vi "IniScrewPara.vi"(8 "error in":errorcluster, 10 "Screw section":string="Info", 11 "INI file path":path=path "D:/ZDX201 塗膠螺絲鎖固自動化_鴻海/ZDX201_LabView/iniData/screw_iniData.ini") -> (0 "data path":path, 1 "Delay":u32, 2 "Screw_L":string="172.100.1.1:1239", 3 "Screw_R":string="172.100.1.22")   [LabVIEW 2019]
uses:
  <vilib>/Utility/config.llb/Read Key (String).vi
  <vilib>/Utility/config.llb/Read Key (U32).vi
  <vilib>/Utility/config.llb/Read Key (Path).vi
  <vilib>/Utility/config.llb/NI_LVConfig.lvlib
panel:
  out "error out":errorcluster
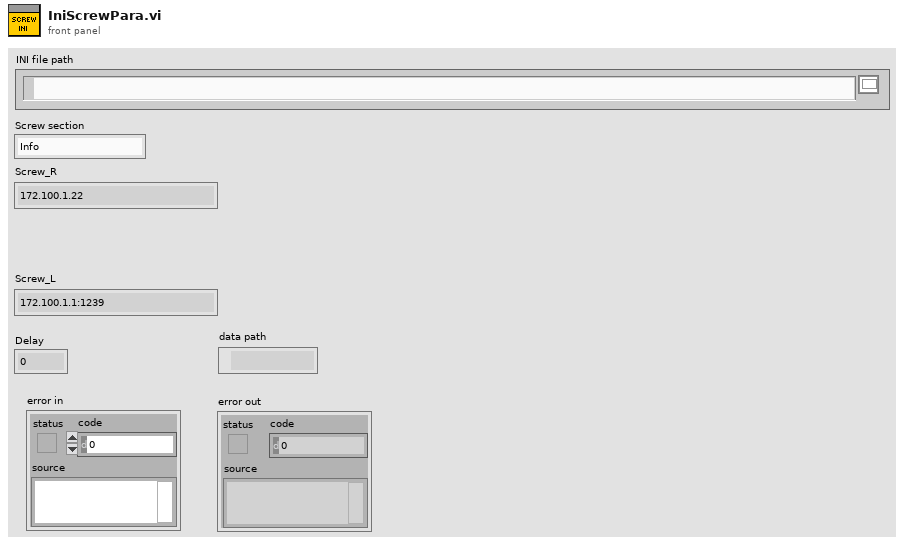
[diagram p1: front panel]
types:
  T1 = typedef "NI_LVConfig.lvlib/Config Data RefNum.ctl" = refnum<k1>
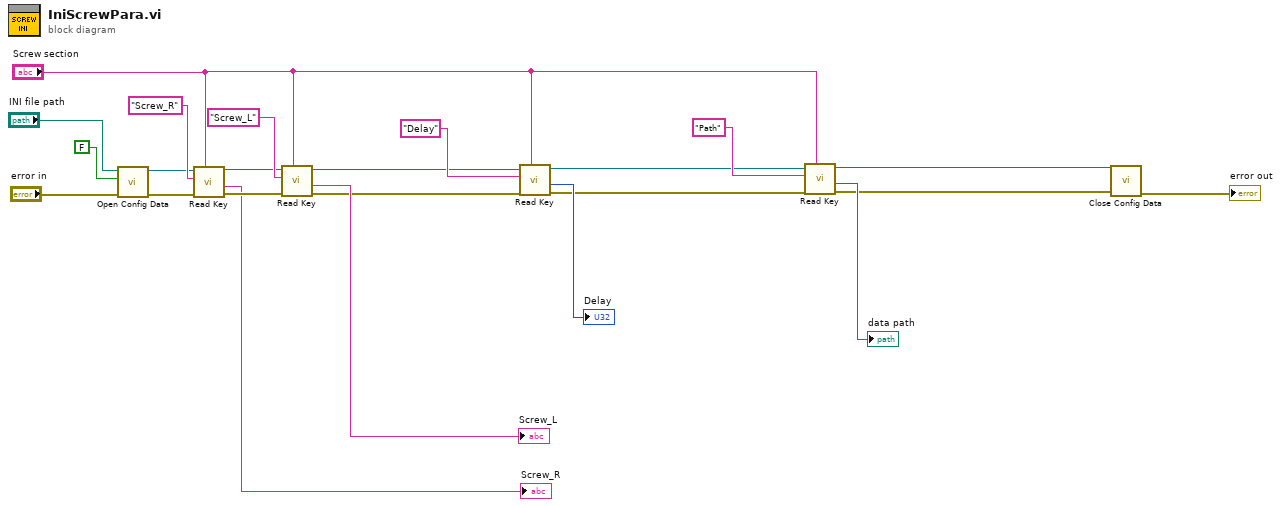
[diagram p0: block diagram]
diagram:
  n1 = call <vilib>:"Open Config Data.vi"("error in (no error)"="error in", "create file if necessary (T)"=FALSE ("create file if necessary? (T)"), "configuration file path"="INI file path") -> ("error out"=w21:errorcluster, "refnum"=w19:T1)  [unwired: 6 in, 1 out]
  n2 = call-poly <vilib>:"Read Key.vi"("section"="Screw section", "error in (no error)"=w21, "key"="Screw_R", "refnum"=w19) -> ("error out"=w14:errorcluster, "value"=→"Screw_R":string, "refnum out"=w15:T1)  [unwired: 2 in, 3 out]
  n3 = call-poly <vilib>:"Read Key.vi"("section"="Screw section", "error in (no error)"=w14, "key"="Screw_L", "refnum"=w15) -> ("error out"=w9:errorcluster, "value"=→"Screw_L":string, "refnum out"=w10:T1)  [unwired: 2 in, 3 out]
  n4 = call-poly <vilib>:"Read Key.vi"("section"="Screw section", "error in (no error)"=w9, "key"="Delay", "refnum"=w10) -> ("error out"=w5:errorcluster, "value"=→"Delay":u32, "refnum out"=w6:T1)  [unwired: 1 in, 4 out]
  n5 = call-poly <vilib>:"Read Key.vi"("section"="Screw section", "error in (no error)"=w5, "key"="Path", "refnum"=w6) -> ("error out"=w2:errorcluster, "value"=→"data path":path, "refnum out"=w1:T1)  [unwired: 1 in, 4 out]
  n6 = call <vilib>:"Close Config Data.vi"("error in (no error)"=w2, "refnum"=w1) -> ("error out"=→"error out":errorcluster)  [unwired: 1 in, 8 out]
